vi "Constructor.vi"() -> (3 "Excel Logger.lvclass":refnum<class "Excel Logger.lvclass">)   [LabVIEW 2016, in "Excel Logger.lvclass"]
uses:
  Excel Logger.lvclass
  Excel Logger.lvclass/Excel Logger.ctl
  Excel Interface/Excel Interface.lvclass
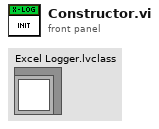
[diagram p1: front panel]
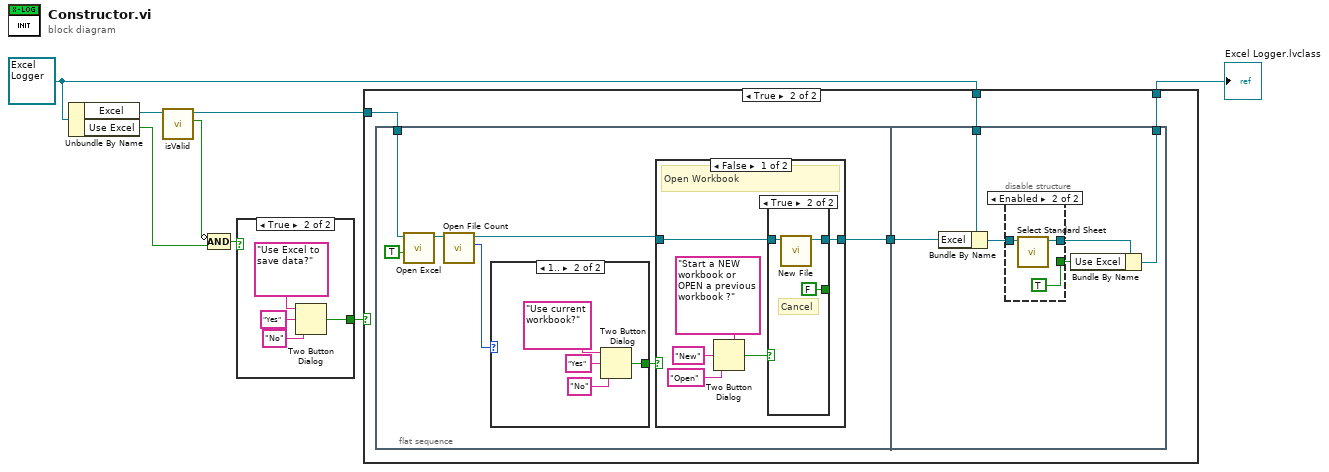
[diagram p0: block diagram]
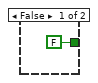
[diagram p2: hidden frame]
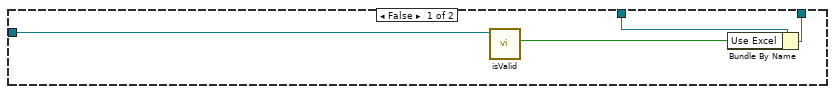
[diagram p3: hidden frame]
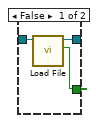
[diagram p4: hidden frame]
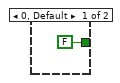
[diagram p6: hidden frame]
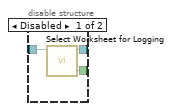
[diagram p7: hidden frame]
diagram:
  w2 = refnum<class "Excel Logger.lvclass"> refnum ("Excel Logger.lvclass")
  n1 = Unbundle By Name(w2) -> ("Excel"=w8:refnum<class "Excel Interface.lvclass">, "Use Excel"=w6:bool)
  n2 = call-dynamic "isValid.vi"("Excel Interface in"=w8) -> ("valid"=w7:bool, "Excel Interface out"=w3:refnum<class "Excel Interface.lvclass">)  [unwired: 8 in, 1 out]
  n3 = Compound Arithmetic op=AND(invert w7, w6) -> (w5:bool)
  n4 = case shown="True" w5 {
    tunnel: [FALSE ("T button?") w10] -> w4
    frame False {
    }
    frame True {
      n5 = Two Button Dialog(message="Use Excel to save data?", 1:"No" ("F button name (\"Cancel\")"), 2:"Yes" ("T button name (\"OK\")")) -> (T button?=w10:bool)
    }
  }
  n6 = case shown="True" w4 {
    tunnel: w3 -> [w15 w21]
    tunnel: w2 -> [w17 w20]
    tunnel: [w16 w19] -> w1
    frame False {
      n7 = call-dynamic "isValid.vi"("Excel Interface in"=w15) -> ("valid"=w14:bool)  [unwired: 8 in, 2 out]
      n8 = Bundle By Name(cluster=w17, "Use Excel"=w14) -> (w16:refnum<class "Excel Logger.lvclass">)
    }
    frame True {
      n9 = flat-sequence {
        tunnel: w21 -> [w28]
        tunnel: [w22] -> w18
        tunnel: w20 -> [w49]
        tunnel: [w51] -> w19
        tunnel: w18 -> [w47]
        frame #0 {
          n10 = call-dynamic "Open Excel.vi"("Visible"=TRUE, "Excel Interface in"=w28) -> ("Excel Interface out"=w27:refnum<class "Excel Interface.lvclass">)  [unwired: 8 in, 1 out]
          n11 = call-dynamic "Open File Count.vi"("Excel Interface in"=w27) -> ("Count"=w26:i32, "Excel Interface out"=w25:refnum<class "Excel Interface.lvclass">)  [unwired: 8 in, 1 out]
          n12 = case shown="1.." w26 {
            tunnel: [FALSE ("T button?") w43] -> w24
            frame 0, Default {
            }
            frame 1.. {
              n13 = Two Button Dialog(message="Use current workbook?", 1:"No" ("F button name (\"Cancel\")"), 2:"Yes" ("T button name (\"OK\")")) -> (T button?=w43:bool)
            }
          }
          n14 = case shown="False" w24 {
            tunnel: w25 -> [w30 w41]
            tunnel: [w29 w41] -> w22
            frame False {
              # "Open Workbook"
              n15 = Two Button Dialog(message="Start a NEW workbook or OPEN a previous workbook ?", 1:"Open" ("F button name (\"Cancel\")"), 2:"New" ("T button name (\"OK\")")) -> (T button?=w31:bool)
              n16 = case shown="True" w31 {
                tunnel: w30 -> [w37 w40]
                tunnel: [w36 w38] -> w29
                tunnel: [w35 FALSE ("cancelled")] -> _
                frame False {
                  n17 = call-dynamic "Load File.vi"("Excel Interface in"=w37) -> ("cancelled"=w35:bool, "Excel Interface out"=w36:refnum<class "Excel Interface.lvclass">)  [unwired: 8 in, 1 out]
                }
                frame True {
                  # "Cancel"
                  n18 = call-dynamic "New File.vi"("Excel Interface in"=w40) -> ("Excel Interface out"=w38:refnum<class "Excel Interface.lvclass">)  [unwired: 9 in, 1 out]
                }
              }
            }
            frame True {
              # "Use already open WB"
            }
          }
        }
        frame #1 {
          n19 = Bundle By Name(cluster=w49, "Excel"=w47) -> (w48:refnum<class "Excel Logger.lvclass">)
          n20 = disable-structure shown="Enabled" {
            disable-tunnel: [w55 w57] -> w52
            disable-tunnel: [w54 TRUE ("Canceled")] -> w50
            disable-tunnel: w48 -> [w53 w58]
            frame Disabled {
              n21 = call "Select Worksheet for Logging.vi"("Excel Logger.lvclass"=w53) -> ("Canceled"=w54:bool, "Excel Logger.lvclass 2"=w55:refnum<class "Excel Logger.lvclass">)  [unwired: 9 in]
            }
            frame Enabled {
              n22 = call-dynamic "Select Standard Sheet.vi"("Excel Logger in"=w58) -> ("Excel Logger out"=w57:refnum<class "Excel Logger.lvclass">)  [unwired: 9 in, 1 out]
            }
          }
          n23 = Bundle By Name(cluster=w52, "Use Excel"=w50) -> (w51:refnum<class "Excel Logger.lvclass">)
        }
      }
    }
  }
  "Excel Logger.lvclass" <- w1
